vi "Struct Fill Cluster By Items Record.vi"(7 "reinit cluster to default (false)":bool, 8 "error in":errorcluster, 9 "data start offset (0)":i32, 10 "data in":u8[](array[numeric])=[9, 0, 0, 0, 15, 0, 0, 0, 1, 78, 0, 1, 0, 0, 0, 1, 0, 0, 0, 1, 0, 0, 0, 43, 0, 0, 0, 1, 97, 3, 1, 0, 0, 0, 4, 0, 0, 0, 0, 0, 0, 0, 0, 0, 240, 63, 0, 0, 0, 0, 0, 0, 0, 64, 0, 0, 0, 0, 0, 0, 8, 64, 0, 0, 0, 0, 0, 0, 16, 64, 43, 0, 0, 0, 1, 66, 3, 2, 0, 0, 0, 2, 0, 0, 0, 0, 0, 0, 0, 0, 0, 240, 63, 0, 0, 0, 0, 0, 0, 8, 64, 0, 0, 0, 0, 0, 0, 0, 64, 0, 0, 0, 0, 0, 0, 16, 64, 22, 0, 0, 0, 3, 115, 116, 114, 4, 1, 0, 0, 0, 9, 0, 0, 0, 100, 118, 101, 32, 104, 111, 118, 110, 111, 44, 0, 0, 0, 2, 99, 97, 131, 2, 0, 0, 0, 1, 0, 0, 0, 0, 0, 0, 0, 0, 0, 240, 63, 0, 0, 0, 0, 0, 0, 240, 63, 0, 0, 0, 0, 0, 0, 0, 64, 0, 0, 0, 0, 0, 0, 240, 191, 109, 0, 0, 0, 5, 115, 116, 114, 117, 99, 5, 1, 0, 0, 0, 1, 0, 0, 0, 3, 0, 0, 0, 16, 0, 0, 0, 3, 115, 116, 114, 4, 1, 0, 0, 0, 3, 0, 0, 0, 97, 115, 115, 19, 0, 0, 0, 1, 110, 3, 1, 0, 0, 0, 1, 0, 0, 0, 0, 0, 0, 0, 0, 128, 75, 64, 43, 0, 0, 0, 1, 65, 3, 2, 0, 0, 0, 2, 0, 0, 0, 0, 0, 0, 0, 0, 0, 240, 63, 0, 0, 0, 0, 0, 0, 8, 64, 0, 0, 0, 0, 0, 0, 0, 64, 0, 0, 0, 0, 0, 0, 16, 64, 218, 0, 0, 0, 2, 115, 118, 5, 1, 0, 0, 0, 2, 0, 0, 0, 3, 0, 0, 0, 16, 0, 0, 0, 3, 115, 116, 114, 4, 1, 0, 0, 0, 3, 0, 0, 0, 97, 115, 115, 19, 0, 0, 0, 1, 110, 3, 1, 0, 0, 0, 1, 0, 0, 0, 0, 0, 0, 0, 0, 128, 75, 64, 43, 0, 0, 0, 1, 65, 3, 2, 0, 0, 0, 2, 0, 0, 0, 0, 0, 0, 0, 0, 0, 240, 63, 0, 0, 0, 0, 0, 0, 8, 64, 0, 0, 0, 0, 0, 0, 0, 64, 0, 0, 0, 0, 0, 0, 16, 64, 3, 0, 0, 0, 34, 0, 0, 0, 3, 115, 116, 114, 4, 1, 0, 0, 0, 21, 0, 0, 0, 110, 101, 106, 97, 107, 101, 106, 32, 106, 105, 110, 101, 106, 32, 114, 101, 116, 101, 122, 101, 99, 19, 0, 0, 0, 1, 110, 3, 1, 0, 0, 0, 1, 0, 0, 0, 0, 0, 0, 0, 0, 0, 86, 64, 43, 0, 0, 0, 1, 65, 3, 2, 0, 0, 0, 2, 0, 0, 0, 0, 0, 0, 0, 0, 0, 240, 63, 0, 0, 0, 0, 0, 0, 8, 64, 0, 0, 0, 0, 0, 0, 0, 64, 0, 0, 0, 0, 0, 0, 16, 64, 132, 1, 0, 0, 2, 115, 99, 5, 2, 0, 0, 0, 2, 0, 0, 0, 3, 0, 0, 0, 16, 0, 0, 0, 3, 115, 116, 114, 4, 1, 0, 0, 0, 3, 0, 0, 0, 97, 115, 115, 19, 0, 0, 0, 1, 110, 3, 1, 0, 0, 0, 1, 0, 0, 0, 0, 0, 0, 0, 0, 128, 75, 64, 43, 0, 0, 0, 1, 65, 3, 2, 0, 0, 0, 2, 0, 0, 0, 0, 0, 0, 0, 0, 0, 240, 63, 0, 0, 0, 0, 0, 0, 8, 64, 0, 0, 0, 0, 0, 0, 0, 64, 0, 0, 0, 0, 0, 0, 16, 64, 3, 0, 0, 0, 16, 0, 0, 0, 3, 115, 116, 114, 4, 1, 0, 0, 0, 3, 0, 0, 0, 97, 115, 115, 19, 0, 0, 0, 1, 110, 3, 1, 0, 0, 0, 1, 0, 0, 0, 0, 0, 0, 0, 0, 128, 75, 64, 43, 0, 0, 0, 1, 65, 3, 2, 0, 0, 0, 2, 0, 0, 0, 0, 0, 0, 0, 0, 0, 240, 63, 0, 0, 0, 0, 0, 0, 8, 64, 0, 0, 0, 0, 0, 0, 0, 64, 0, 0, 0, 0, 0, 0, 16, 64, 3, 0, 0, 0, 16, 0, 0, 0, 3, 115, 116, 114, 4, 1, 0, 0, 0, 3, 0, 0, 0, 97, 115, 115, 19, 0, 0, 0, 1, 110, 3, 1, 0, 0, 0, 1, 0, 0, 0, 0, 0, 0, 0, 0, 128, 75, 64, 43, 0, 0, 0, 1, 65, 3, 2, 0, 0, 0, 2, 0, 0, 0, 0, 0, 0, 0, 0, 0, 240, 63, 0, 0, 0, 0, 0, 0, 8, 64, 0, 0, 0, 0, 0, 0, 0, 64, 0, 0, 0, 0, 0, 0, 16, 64, 3, 0, 0, 0, 16, 0, 0, 0, 3, 115, 116, 114, 4, 1, 0, 0, 0, 3, 0, 0, 0, 97, 115, 115, 19, 0, 0, 0, 1, 110, 3, 1, 0, 0, 0, 1, 0, 0, 0, 0, 0, 0, 0, 0, 128, 75, 64, 43, 0, 0, 0, 1, 65, 3, 2, 0, 0, 0, 2, 0, 0, 0, 0, 0, 0, 0, 0, 0, 240, 63, 0, 0, 0, 0, 0, 0, 8, 64, 0, 0, 0, 0, 0, 0, 0, 64, 0, 0, 0, 0, 0, 0, 16, 64, 26, 0, 0, 0, 4, 99, 115, 116, 114, 5, 1, 0, 0, 0, 3, 0, 0, 0, 0, 0, 0, 0, 0, 0, 0, 0, 0, 0, 0, 0], 11 "cluster ref (empty)":refnum<vi>) -> (0 "error out":errorcluster, 2 "octave struct out":T1[](array[typedef]), 3 "cluster ref out (copy)":refnum<vi>)   [LabVIEW 2013, in "GOLPI library.lvlib"]
doc: "This VI will use binary struct data generated by GNU Octave GOLPI function 'golpi_conv_struct()'. It will try to assign all elements from the Octave to the elements of matching names in the referenced cluser. Optionally it can reset the cluster default before. If it is called with invalid reference to the cluster it will just parse the binary data and return the items list. The function is recoursive so it should be able to assign clusters within clusters and so on."
uses:
  GOLPI library.lvlib
  Type Definitions/Struct Item Record.ctl
  Type Definitions/Struct Item Types.ctl
  Type Definitions/Custom Error Codes Enum Type Def.vi
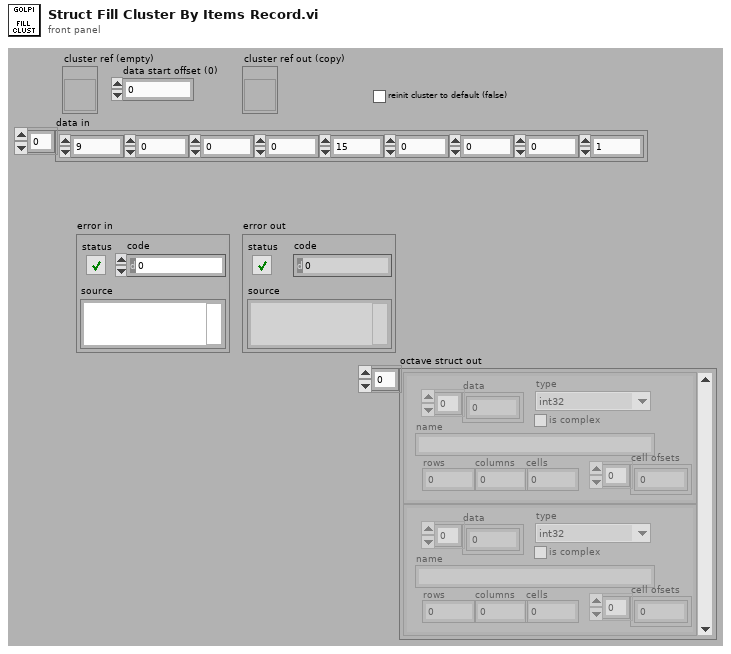
[diagram p1: front panel]
types:
  T1 = typedef "GOLPI library.lvlib/Struct Item Record.ctl" = cluster{"data":u8[], "type":T2, "name":string, "rows":i32, "columns":i32, "cells":i32, "is complex":bool, "cell ofsets":u32[]}
  T2 = typedef "GOLPI library.lvlib/Struct Item Types.ctl" = enum16{"int32", "uint32", "single", "double", "string", "cell array"}
  T3 = typedef "GOLPI library.lvlib/Custom Error Codes Enum Type Def.vi" = enum16{"no error", "00 working directory PAR1 missing", "01 octave binary PAR1 missing", "02 octave report error PAR1", "03 empty output last cmd PAR1", "04 missing temporary file PAR1", "05 pwd PAR 1 not exist", "06 oct package not installed", "10 var PAR1 not string, vect", "11 var PAR1 not num, scal, ~compl", "12 var PAR1 not num, scal, compl", "13 var PAR1 not num, vect, ~compl", "14 var PAR1 not num, vect, compl", "15 var PAR1 not num, mat, ~compl", "16 var PAR1 not num, mat, ~compl", "30 read timeout", "60 bitstream transport failed", "61 bitstream decode error PAR1", "62 bitstream cannot be set", "70 struct transfer not possible", "80 struct: cluster elem. PAR1 not implem.", "81 struct: structure field PAR1 not implem.", "82 struct: size mismatch of PAR1", "83 struct: type mismatch of PAR1", "98 internal error", "99 not finished"}
  T4 = enum16{"big-endian, network order", "native, host order", "little-endian"}
  T5 = typedef "GOLPI library.lvlib/Struct Data Types.ctl" = enum16{"n/a", "Real", "Complex", "String/path", "Cluster", "Bool"}
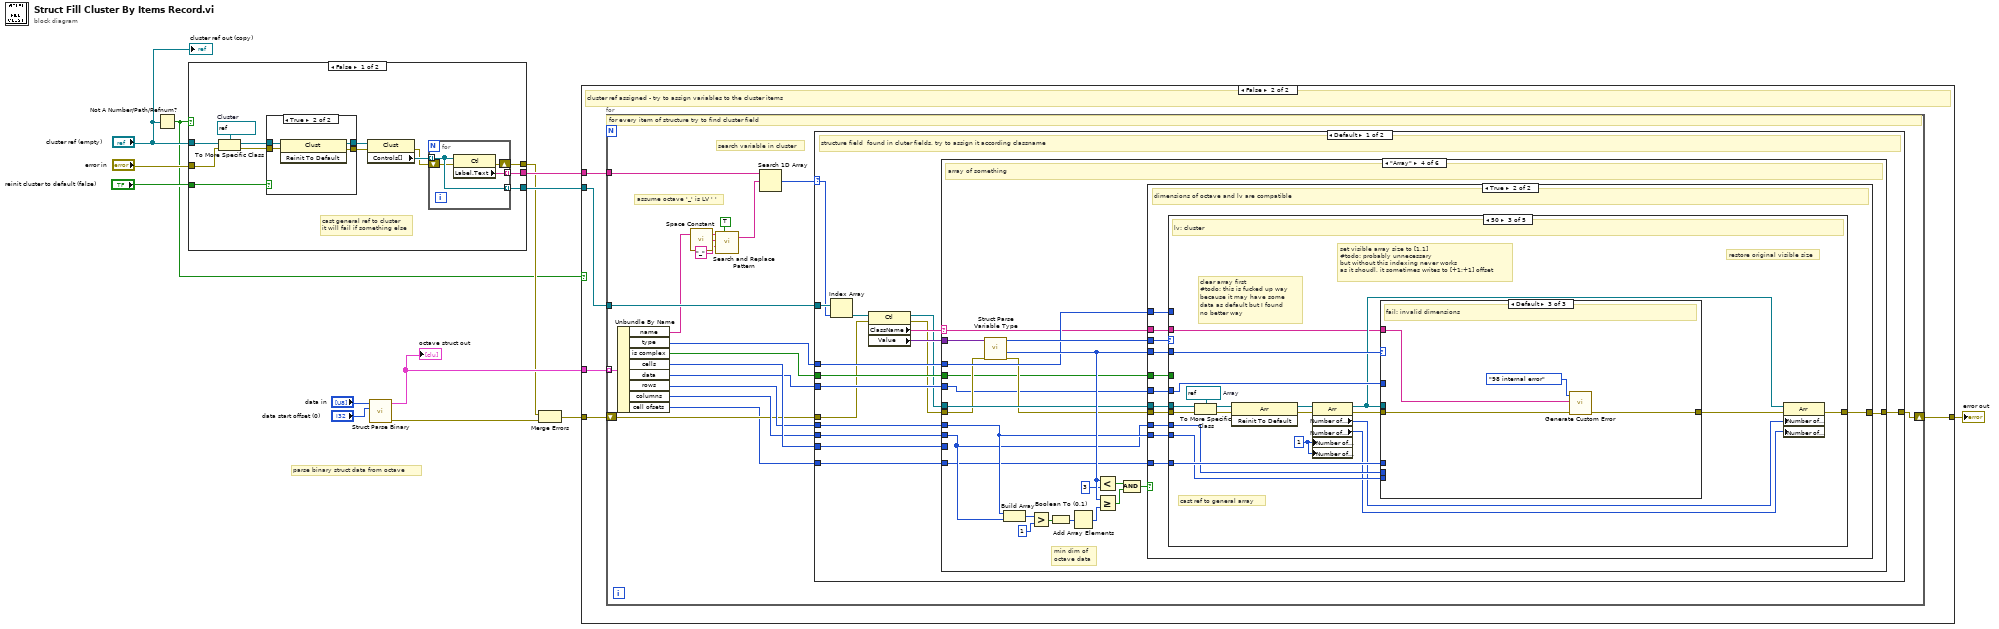
[diagram p0: block diagram]
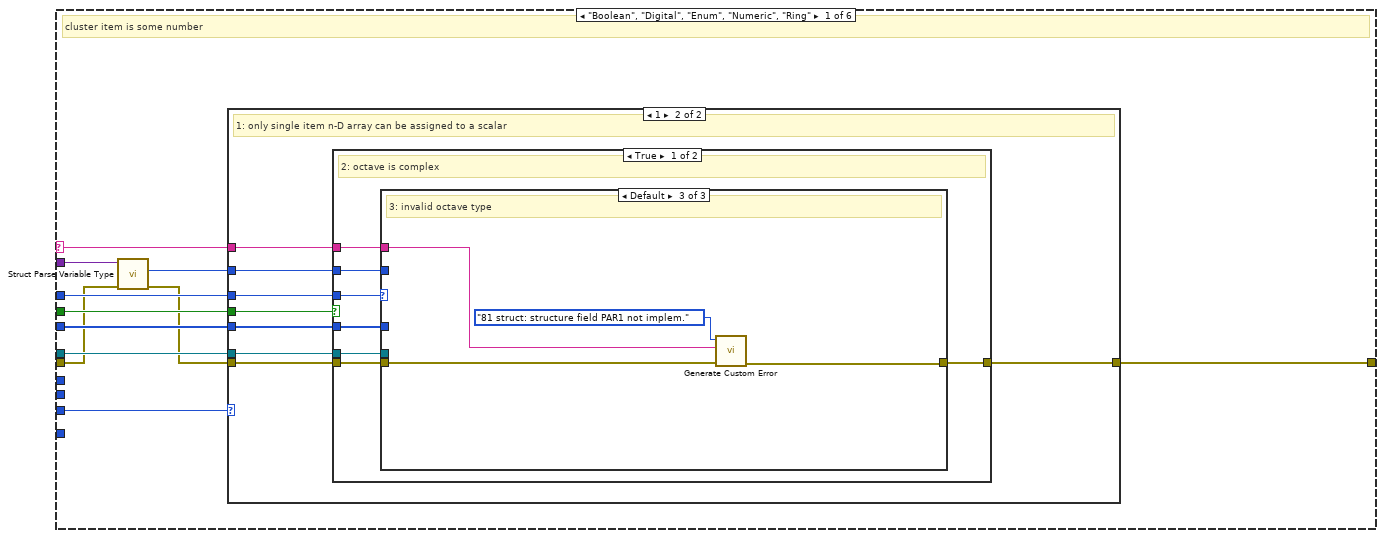
[diagram p3: hidden frame]
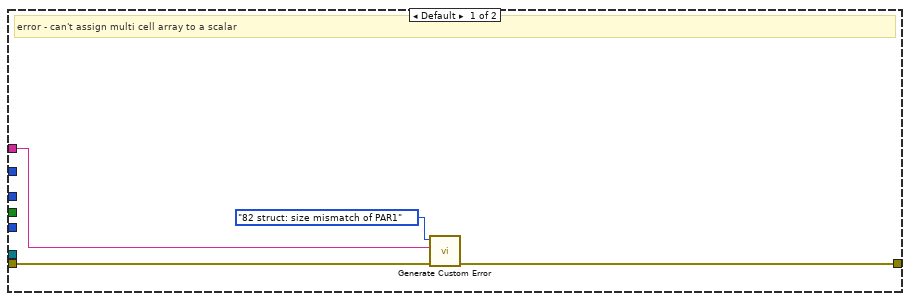
[diagram p4: hidden frame]
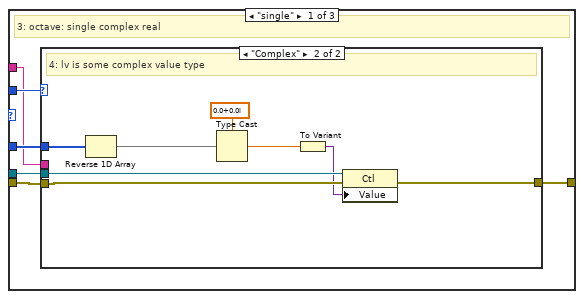
[diagram p5: hidden frame]
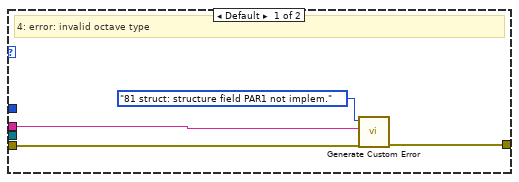
[diagram p6: hidden frame]
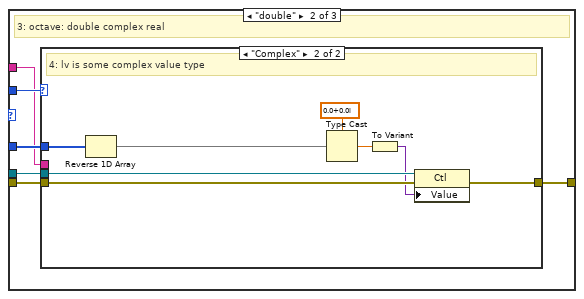
[diagram p7: hidden frame]
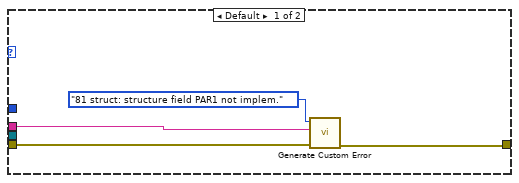
[diagram p8: hidden frame]
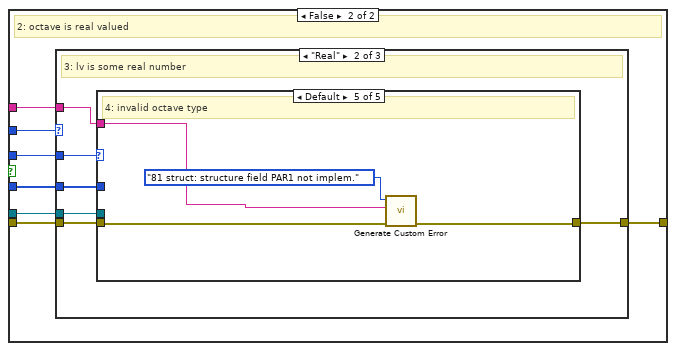
[diagram p9: hidden frame]
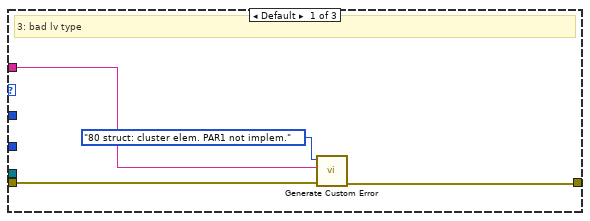
[diagram p10: hidden frame]
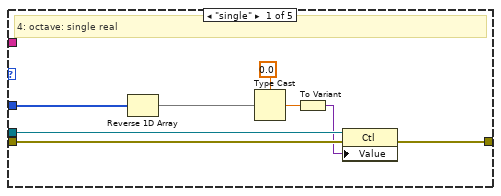
[diagram p11: hidden frame]
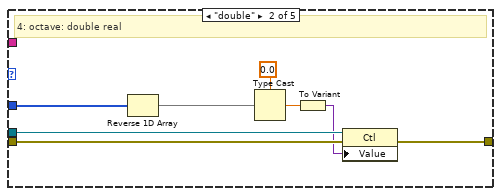
[diagram p12: hidden frame]
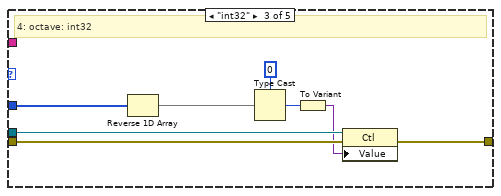
[diagram p13: hidden frame]
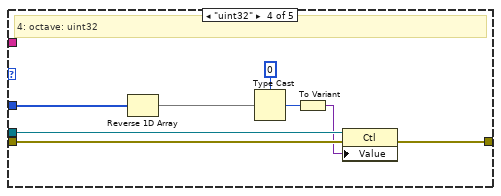
[diagram p14: hidden frame]
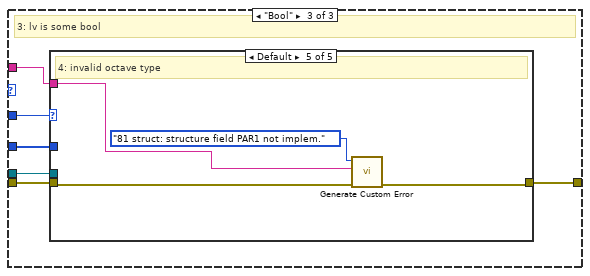
[diagram p15: hidden frame]
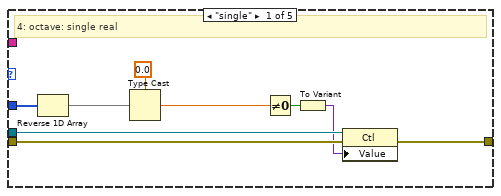
[diagram p16: hidden frame]
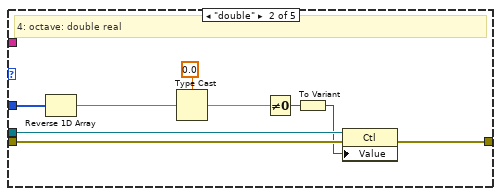
[diagram p17: hidden frame]
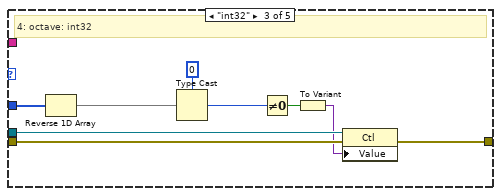
[diagram p18: hidden frame]
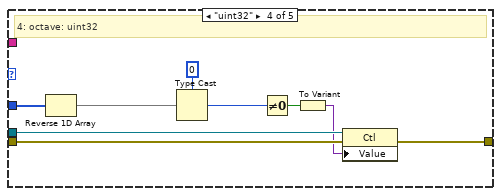
[diagram p19: hidden frame]
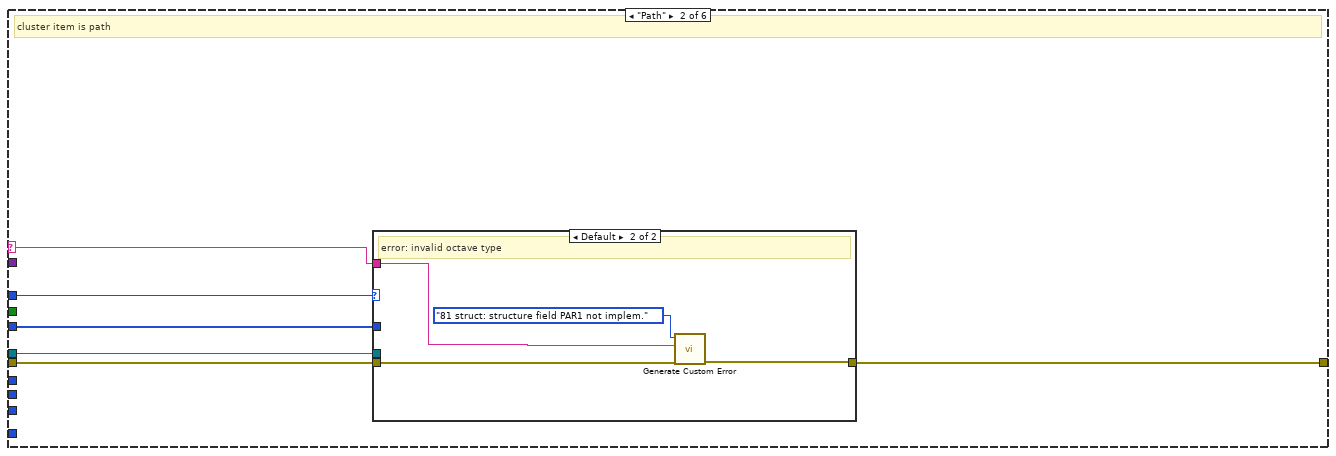
[diagram p20: hidden frame]
diagram:
  # "parse binary struct data from octave"
  n1 = Not A Number/Path/Refnum?(number/path/refnum="cluster ref (empty)") -> (NaN/Path/Refnum?=w1:bool)
  n2 = case shown="False" w1 {
    tunnel: [w25 _] -> w11
    tunnel: [w24 _] -> w10
    tunnel: "error in" -> [w22 w37]
    tunnel: "cluster ref (empty)" -> [w15 _]
    tunnel: "reinit cluster to default (false)" -> [w17 _]
    tunnel: [w14 w37] -> w4
    frame False {
      w23 = refnum<vi> refnum  # Cluster
      # "cast general ref to cluster\nit will fail if something else"
      n3 = To More Specific Class(target class=w23, reference=w15, error in=w22) -> (specific class reference=w19:refnum<vi>, error out=w18:errorcluster)
      n4 = case shown="True" w17 {
        tunnel: [w28 w32] -> w21
        tunnel: [w27 w31] -> w20
        tunnel: w19 -> [w27 w30]
        tunnel: w18 -> [w28 w29]
        frame False {
        }
        frame True {
          n5 = invoke class="Clust" method="Reinit To Default"(reference=w30, error in=w29) -> (reference out=w31:refnum<vi>, error out=w32:errorcluster)  [unwired: 1 in, 1 out]
        }
      }
      n6 = property class="Clust"(reference=w20, error in=w21) -> (error out=w16:errorcluster, "Controls[]"=w26:refnum<vi>[])  [unwired: 1 out]
      n7 = for {
        tunnel: w26 -> [w35] mode=indexing
        tunnel: [w36] -> w25 mode=indexing
        tunnel: [w35] -> w24 mode=indexing
        shift-right: [w33] -> w14
        shift-left: w16 -> [w34]
        n8 = property class="Ctl"(reference=w35, error in=w34) -> (error out=w33:errorcluster, "Label.Text"=w36:string)  [unwired: 1 out]
      }
    }
    frame True {
    }
  }
  n9 = call "Struct Parse Binary.vi"("data start offset (0)"="data start offset (0)", "data in"="data in") -> ("error out"=w3:errorcluster, "struct items"=w12:T1[])  [unwired: 8 in]
  "octave struct out" <- w12
  n10 = Merge Errors(w4, w3) -> (w2:errorcluster)
  n11 = case shown="False" w1 {
    tunnel: w12 -> [_ w43]
    tunnel: w11 -> [_ w42]
    tunnel: w10 -> [_ w41]
    tunnel: [w38 w40] -> w9
    tunnel: w2 -> [w38 w39]
    frame True {
      # "no cluster ref assigned - skip assigning, just parse struct"
    }
    frame False {
      # "cluster ref assigned - try to assign variables to the cluster items"
      n12 = for {
        tunnel: w43 -> [w61] mode=indexing
        tunnel: w42 -> [w60]
        tunnel: w41 -> [w59]
        shift-right: [w52] -> w40
        shift-left: w39 -> [w51]
        # "assume octave '_' is LV ' '"
        # "search variable in cluster"
        # "for every item of structure try to find cluster field"
        n13 = Unbundle By Name(w61) -> ("name"=w48:string, "type"=w58:T2, "is complex"=w57:bool, "cells"=w56:i32, "data"=w55:u8[], "rows"=w54:i32, "columns"=w53:i32, "cell ofsets"=w50:u32[])
        n14 = call <vilib>:"Space Constant.vi"() -> ("String"=w44:string)
        n15 = call <vilib>:"Search and Replace Pattern.vi"("string"=w48, "regular expression (\"\")"="_", "replace string (\"\")"=w44, "replace all? (F)"=TRUE) -> ("result string"=w47:string)  [unwired: 1 in, 1 out]
        n16 = Search 1D Array(1D array=w60, element=w47) -> (index of element=w49:i32)  [unwired: 1 in]
        n17 = case shown="Default" w49 {
          selector: w49 -> [w76 _]
          tunnel: w59 -> [w77 _]
          tunnel: w58 -> [w72 _]
          tunnel: w57 -> [w71 _]
          tunnel: w56 -> [w70 _]
          tunnel: w55 -> [w69 _]
          tunnel: w54 -> [w66 _]
          tunnel: w53 -> [w65 _]
          tunnel: [w64 w696] -> w52
          tunnel: w51 -> [w63 w696]
          tunnel: w50 -> [w62 _]
          frame Default {
            # "structure field  found in cluter fields, try to assign it according classname"
            n18 = Index Array(array=w77, index=w76) -> (element=w75:refnum<vi>)
            n19 = property class="Ctl"(reference=w75, error in=w63) -> (reference out=w68:refnum<vi>, error out=w67:errorcluster, "ClassName"=w74:string, "Value"=w73:variant)
            n20 = case shown="\"Array\"" w74 {
              selector: w74 -> [w78 w247 w264 w280 _ w694]
              tunnel: w73 -> [w88 _ _ w282 _ _]
              tunnel: w72 -> [w87 w252 w269 w289 w678 _]
              tunnel: w71 -> [w83 _ _ w286 _ _]
              tunnel: w70 -> [w84 _ _ _ w680 _]
              tunnel: w69 -> [w86 w251 w268 w285 w672 _]
              tunnel: w68 -> [w82 w250 w267 w291 w673 _]
              tunnel: w67 -> [w80 w249 w266 w288 w681 w693]
              tunnel: [w81 w248 w265 w292 w671 w692] -> w64
              tunnel: w66 -> [_ _ _ w284 _ _]
              tunnel: w65 -> [_ _ _ w283 _ _]
              tunnel: w62 -> [_ _ _ w281 _ _]
              frame "Boolean", "Digital", "Enum", "Numeric", "Ring" {
                # "cluster item is some number"
                n21 = call "Struct Parse Variable Type.vi"("error in"=w80, "variant in"=w88) -> ("error out"=w79:errorcluster, "data type"=w85:T5)  [unwired: 6 in, 2 out]
                n22 = case shown="1" w84 {
                  tunnel: w87 -> [_ w100]
                  tunnel: w86 -> [_ w99]
                  tunnel: w85 -> [_ w98]
                  tunnel: w83 -> [_ w97]
                  tunnel: w82 -> [_ w96]
                  tunnel: w79 -> [w91 w95]
                  tunnel: [w90 w94] -> w81
                  tunnel: w78 -> [w89 w93]
                  frame Default {
                    # "error - can't assign multi cell array to a scalar"
                    n23 = call "Generate Custom Error.vi"("error in"=w91, "PAR1"=w89, "GOLPI error"=Custom_Error_Codes_Enum_Type_Def.vi."82 struct: size mismatch of PAR1") -> ("error out"=w90:errorcluster)  [unwired: 8 in]
                  }
                  frame 1 {
                    # "1: only single item n-D array can be assigned to a scalar"
                    n24 = case shown="True" w97 {
                      tunnel: w100 -> [w107 w154]
                      tunnel: w99 -> [w106 w153]
                      tunnel: w98 -> [w105 w149]
                      tunnel: w96 -> [w104 w152]
                      tunnel: w95 -> [w103 w151]
                      tunnel: [w102 w150] -> w94
                      tunnel: w93 -> [w101 w148]
                      frame True {
                        # "2: octave is complex"
                        n25 = case shown="Default" w107 {
                          tunnel: w106 -> [w112 w130 _]
                          tunnel: w105 -> [w113 w131 _]
                          tunnel: w104 -> [w111 w129 _]
                          tunnel: w103 -> [w110 w128 w146]
                          tunnel: [w109 w127 w145] -> w102
                          tunnel: w101 -> [w108 w126 w144]
                          frame "single" {
                            # "3: octave: single complex real"
                            n26 = case shown="\"Complex\"" w113 {
                              tunnel: w112 -> [_ w125]
                              tunnel: w111 -> [_ w122]
                              tunnel: w110 -> [w116 w121]
                              tunnel: [w115 w118] -> w109
                              tunnel: w108 -> [w114 _]
                              frame Default {
                                # "4: error: invalid octave type"
                                n27 = call "Generate Custom Error.vi"("error in"=w116, "PAR1"=w114, "GOLPI error"=Custom_Error_Codes_Enum_Type_Def.vi."81 struct: structure field PAR1 not implem.") -> ("error out"=w115:errorcluster)  [unwired: 8 in]
                              }
                              frame "Complex" {
                                # "4: lv is some complex value type"
                                n28 = Reverse 1D Array(array=w125) -> (reversed array=w124:u8[])
                                n29 = Type Cast(type=csg 0.0+0.0i, x=w124) -> (*(type *) &x=w120:csg)
                                n30 = To Variant(anything=w120) -> (Variant=w119:variant)
                                n31 = property class="Ctl"(reference=w122, error in=w121, "Value"=w119) -> (error out=w118:errorcluster)  [unwired: 1 out]
                              }
                            }
                          }
                          frame "double" {
                            # "3: octave: double complex real"
                            n32 = case shown="\"Complex\"" w131 {
                              tunnel: w130 -> [_ w143]
                              tunnel: w129 -> [_ w140]
                              tunnel: w128 -> [w134 w139]
                              tunnel: [w133 w136] -> w127
                              tunnel: w126 -> [w132 _]
                              frame Default {
                                n33 = call "Generate Custom Error.vi"("error in"=w134, "PAR1"=w132, "GOLPI error"=Custom_Error_Codes_Enum_Type_Def.vi."81 struct: structure field PAR1 not implem.") -> ("error out"=w133:errorcluster)  [unwired: 8 in]
                              }
                              frame "Complex" {
                                # "4: lv is some complex value type"
                                n34 = Reverse 1D Array(array=w143) -> (reversed array=w142:u8[])
                                n35 = Type Cast(type=cdb 0.0+0.0i, x=w142) -> (*(type *) &x=w138:cdb)
                                n36 = To Variant(anything=w138) -> (Variant=w137:variant)
                                n37 = property class="Ctl"(reference=w140, error in=w139, "Value"=w137) -> (error out=w136:errorcluster)  [unwired: 1 out]
                              }
                            }
                          }
                          frame Default {
                            # "3: invalid octave type"
                            n38 = call "Generate Custom Error.vi"("error in"=w146, "PAR1"=w144, "GOLPI error"=Custom_Error_Codes_Enum_Type_Def.vi."81 struct: structure field PAR1 not implem.") -> ("error out"=w145:errorcluster)  [unwired: 8 in]
                          }
                        }
                      }
                      frame False {
                        # "2: octave is real valued"
                        n39 = case shown="\"Real\"" w149 {
                          tunnel: w154 -> [_ w164 w206]
                          tunnel: w153 -> [_ w163 w205]
                          tunnel: w152 -> [_ w162 w204]
                          tunnel: w151 -> [w157 w161 w203]
                          tunnel: [w156 w160 w202] -> w150
                          tunnel: w148 -> [w155 w159 w201]
                          frame Default {
                            # "3: bad lv type"
                            n40 = call "Generate Custom Error.vi"("error in"=w157, "PAR1"=w155, "GOLPI error"=Custom_Error_Codes_Enum_Type_Def.vi."80 struct: cluster elem. PAR1 not implem.") -> ("error out"=w156:errorcluster)  [unwired: 8 in]
                          }
                          frame "Real" {
                            # "3: lv is some real number"
                            n41 = case shown="Default" w164 {
                              tunnel: w163 -> [w172 w180 w188 w196 _]
                              tunnel: w162 -> [w171 w179 w187 w195 _]
                              tunnel: w161 -> [w170 w178 w186 w194 w199]
                              tunnel: [w169 w177 w185 w193 w198] -> w160
                              tunnel: w159 -> [_ _ _ _ w197]
                              frame "single" {
                                # "4: octave: single real"
                                n42 = Reverse 1D Array(array=w172) -> (reversed array=w168:u8[])
                                n43 = Type Cast(type=sgl 0.0, x=w168) -> (*(type *) &x=w166:sgl)
                                n44 = To Variant(anything=w166) -> (Variant=w165:variant)
                                n45 = property class="Ctl"(reference=w171, error in=w170, "Value"=w165) -> (error out=w169:errorcluster)  [unwired: 1 out]
                              }
                              frame "double" {
                                # "4: octave: double real"
                                n46 = Reverse 1D Array(array=w180) -> (reversed array=w176:u8[])
                                n47 = Type Cast(type=0.0, x=w176) -> (*(type *) &x=w174:dbl)
                                n48 = To Variant(anything=w174) -> (Variant=w173:variant)
                                n49 = property class="Ctl"(reference=w179, error in=w178, "Value"=w173) -> (error out=w177:errorcluster)  [unwired: 1 out]
                              }
                              frame "int32" {
                                # "4: octave: int32"
                                n50 = Reverse 1D Array(array=w188) -> (reversed array=w184:u8[])
                                n51 = Type Cast(type=0, x=w184) -> (*(type *) &x=w182:i32)
                                n52 = To Variant(anything=w182) -> (Variant=w181:variant)
                                n53 = property class="Ctl"(reference=w187, error in=w186, "Value"=w181) -> (error out=w185:errorcluster)  [unwired: 1 out]
                              }
                              frame "uint32" {
                                # "4: octave: uint32"
                                n54 = Reverse 1D Array(array=w196) -> (reversed array=w192:u8[])
                                n55 = Type Cast(type=u32 0, x=w192) -> (*(type *) &x=w190:u32)
                                n56 = To Variant(anything=w190) -> (Variant=w189:variant)
                                n57 = property class="Ctl"(reference=w195, error in=w194, "Value"=w189) -> (error out=w193:errorcluster)  [unwired: 1 out]
                              }
                              frame Default {
                                # "4: invalid octave type"
                                n58 = call "Generate Custom Error.vi"("error in"=w199, "PAR1"=w197, "GOLPI error"=Custom_Error_Codes_Enum_Type_Def.vi."81 struct: structure field PAR1 not implem.") -> ("error out"=w198:errorcluster)  [unwired: 8 in]
                              }
                            }
                          }
                          frame "Bool" {
                            # "3: lv is some bool"
                            n59 = case shown="Default" w206 {
                              tunnel: w205 -> [w215 w224 w233 w242 _]
                              tunnel: w204 -> [w214 w223 w232 w241 _]
                              tunnel: w203 -> [w213 w222 w231 w240 w245]
                              tunnel: [w212 w221 w230 w239 w244] -> w202
                              tunnel: w201 -> [_ _ _ _ w243]
                              frame "single" {
                                # "4: octave: single real"
                                n60 = Reverse 1D Array(array=w215) -> (reversed array=w211:u8[])
                                n61 = Type Cast(type=sgl 0.0, x=w211) -> (*(type *) &x=w209:sgl)
                                n62 = Not Equal To 0?(x=w209) -> (x != 0?=w207:bool)
                                n63 = To Variant(anything=w207) -> (Variant=w208:variant)
                                n64 = property class="Ctl"(reference=w214, error in=w213, "Value"=w208) -> (error out=w212:errorcluster)  [unwired: 1 out]
                              }
                              frame "double" {
                                # "4: octave: double real"
                                n65 = Reverse 1D Array(array=w224) -> (reversed array=w220:u8[])
                                n66 = Type Cast(type=0.0, x=w220) -> (*(type *) &x=w218:dbl)
                                n67 = Not Equal To 0?(x=w218) -> (x != 0?=w216:bool)
                                n68 = To Variant(anything=w216) -> (Variant=w217:variant)
                                n69 = property class="Ctl"(reference=w223, error in=w222, "Value"=w217) -> (error out=w221:errorcluster)  [unwired: 1 out]
                              }
                              frame "int32" {
                                # "4: octave: int32"
                                n70 = Reverse 1D Array(array=w233) -> (reversed array=w229:u8[])
                                n71 = Type Cast(type=0, x=w229) -> (*(type *) &x=w227:i32)
                                n72 = Not Equal To 0?(x=w227) -> (x != 0?=w225:bool)
                                n73 = To Variant(anything=w225) -> (Variant=w226:variant)
                                n74 = property class="Ctl"(reference=w232, error in=w231, "Value"=w226) -> (error out=w230:errorcluster)  [unwired: 1 out]
                              }
                              frame "uint32" {
                                # "4: octave: uint32"
                                n75 = Reverse 1D Array(array=w242) -> (reversed array=w238:u8[])
                                n76 = Type Cast(type=u32 0, x=w238) -> (*(type *) &x=w236:u32)
                                n77 = Not Equal To 0?(x=w236) -> (x != 0?=w234:bool)
                                n78 = To Variant(anything=w234) -> (Variant=w235:variant)
                                n79 = property class="Ctl"(reference=w241, error in=w240, "Value"=w235) -> (error out=w239:errorcluster)  [unwired: 1 out]
                              }
                              frame Default {
                                # "4: invalid octave type"
                                n80 = call "Generate Custom Error.vi"("error in"=w245, "PAR1"=w243, "GOLPI error"=Custom_Error_Codes_Enum_Type_Def.vi."81 struct: structure field PAR1 not implem.") -> ("error out"=w244:errorcluster)  [unwired: 8 in]
                              }
                            }
                          }
                        }
                      }
                    }
                  }
                }
              }
              frame "Path" {
                # "cluster item is path"
                n81 = case shown="Default" w252 {
                  tunnel: w251 -> [w255 _]
                  tunnel: w250 -> [w259 _]
                  tunnel: w249 -> [w258 w262]
                  tunnel: [w257 w261] -> w248
                  tunnel: w247 -> [_ w260]
                  frame "string" {
                    # "octave: string"
                    n82 = Byte Array To String(unsigned byte array=w255) -> (string=w254:string)
                    n83 = String To Path(string=w254) -> (path=w253:path)
                    n84 = To Variant(anything=w253) -> (Variant=w256:variant)
                    n85 = property class="Ctl"(reference=w259, error in=w258, "Value"=w256) -> (error out=w257:errorcluster)  [unwired: 1 out]
                  }
                  frame Default {
                    # "error: invalid octave type"
                    n86 = call "Generate Custom Error.vi"("error in"=w262, "PAR1"=w260, "GOLPI error"=Custom_Error_Codes_Enum_Type_Def.vi."81 struct: structure field PAR1 not implem.") -> ("error out"=w261:errorcluster)  [unwired: 8 in]
                  }
                }
              }
              frame "ComboBox", "DAQmxName", "IVILogicalName", "IVIResourceName", "String", "VISAResourceName" {
                # "cluster item is some string type"
                n87 = case shown="Default" w269 {
                  tunnel: w268 -> [w271 _]
                  tunnel: w267 -> [w275 _]
                  tunnel: w266 -> [w274 w278]
                  tunnel: [w273 w277] -> w265
                  tunnel: w264 -> [_ w276]
                  frame "string" {
                    # "octave: string"
                    n88 = Byte Array To String(unsigned byte array=w271) -> (string=w270:string)
                    n89 = To Variant(anything=w270) -> (Variant=w272:variant)
                    n90 = property class="Ctl"(reference=w275, error in=w274, "Value"=w272) -> (error out=w273:errorcluster)  [unwired: 1 out]
                  }
                  frame Default {
                    # "error: invalid octave type"
                    n91 = call "Generate Custom Error.vi"("error in"=w278, "PAR1"=w276, "GOLPI error"=Custom_Error_Codes_Enum_Type_Def.vi."81 struct: structure field PAR1 not implem.") -> ("error out"=w277:errorcluster)  [unwired: 8 in]
                  }
                }
              }
              frame "Array" {
                # "min dim of\noctave data"
                # "array of something"
                n92 = call "Struct Parse Variable Type.vi"("error in"=w288, "variant in"=w282) -> ("error out"=w287:errorcluster, "array dims"=w297:i16, "type id"=w290:i16)  [unwired: 6 in, 1 out]
                n93 = Build Array(w284, w283) -> (w302:i32[])
                n94 = Greater?(x=w302, y=1) -> (0:w300:bool[])
                n95 = Boolean To (0,1)(Boolean=w300) -> (0, 1=w299:i16[])
                n96 = Add Array Elements(numeric array=w299) -> (sum=w298:i16)
                n97 = Less?(x=w297, y=i16 3) -> (x < y?=w295:bool)
                n98 = Greater Or Equal?(x=w297, y=w298) -> (x >= y?=w294:bool)
                n99 = Compound Arithmetic op=AND(w295, w294) -> (w293:bool)
                n100 = case shown="True" w293 {
                  tunnel: w290 -> [_ w318]
                  tunnel: w297 -> [_ w317]
                  tunnel: [w304 w311] -> w292
                  tunnel: w287 -> [w305 w315]
                  tunnel: w291 -> [_ w314]
                  tunnel: w289 -> [_ w316]
                  tunnel: w286 -> [_ w313]
                  tunnel: w285 -> [_ w312]
                  tunnel: w283 -> [_ w310]
                  tunnel: w284 -> [_ w309]
                  tunnel: w281 -> [_ w308]
                  tunnel: w280 -> [w303 w307]
                  frame False {
                    # "incompatible lv and octave dims"
                    n101 = call "Generate Custom Error.vi"("error in"=w305, "PAR1"=w303, "GOLPI error"=Custom_Error_Codes_Enum_Type_Def.vi."82 struct: size mismatch of PAR1") -> ("error out"=w304:errorcluster)  [unwired: 8 in]
                  }
                  frame True {
                    # "dimensions of octave and lv are compatible"
                    n102 = case shown="50" w318 {
                      selector: w318 -> [_ _ _ w575 _]
                      tunnel: w317 -> [w322 w437 w510 w581 _]
                      tunnel: w316 -> [w328 w443 _ _ _]
                      tunnel: w315 -> [w327 w442 w523 w585 w668]
                      tunnel: w314 -> [w326 w441 w524 w586 _]
                      tunnel: w313 -> [w325 w440 _ _ _]
                      tunnel: w312 -> [w324 w439 w521 w583 _]
                      tunnel: [w323 w438 w511 w574 w669] -> w311
                      tunnel: w310 -> [w321 w436 w518 w578 _]
                      tunnel: w309 -> [w320 w435 w519 w577 _]
                      tunnel: w308 -> [_ _ w520 w582 _]
                      tunnel: w307 -> [w319 w434 w505 _ w667]
                      frame 1..11, 21..23 {
                        # "lv: real numerics"
                        n103 = case shown="False" w325 {
                          tunnel: w328 -> [w337 _]
                          tunnel: w327 -> [w336 w432]
                          tunnel: w326 -> [w333 _]
                          tunnel: w324 -> [w335 _]
                          tunnel: [w334 w431] -> w323
                          tunnel: w322 -> [w332 _]
                          tunnel: w321 -> [w331 _]
                          tunnel: w320 -> [w330 _]
                          tunnel: w319 -> [w329 w430]
                          frame False {
                            # "octave: real"
                            n104 = case shown="Default" w337 {
                              tunnel: w336 -> [w340 w362 w384 w406 w428]
                              tunnel: w335 -> [w339 w361 w383 w405 _]
                              tunnel: [w347 w369 w391 w413 w427] -> w334
                              tunnel: w333 -> [w348 w370 w392 w414 _]
                              tunnel: w332 -> [w345 w367 w389 w411 _]
                              tunnel: w331 -> [w343 w365 w387 w409 _]
                              tunnel: w330 -> [w342 w364 w386 w408 _]
                              tunnel: w329 -> [_ _ _ _ w426]
                              frame "int32" {
                                # "octave: int32 array"
                                n105 = Byte Array To String(unsigned byte array=w339) -> (string=w338:string)
                                n106 = Unflatten From String(type=i32[] [], binary string=w338, data includes array or string size? (T)=FALSE ("prepend array or string size? (T)"), byte order (0:big-endian, network order)=T4."little-endian", error in (no error)=w340) -> (value=w346:i32[], error out=w349:errorcluster)  [unwired: 1 out]
                                n107 = case shown="2" w345 {
                                tunnel: w346 -> [w352 w359]
                                tunnel: [w353 w357] -> w344
                                tunnel: w343 -> [_ w356]
                                tunnel: w342 -> [_ w355]
                                frame Default {
                                # "1D"
                                n108 = To Variant(anything=w352) -> (Variant=w353:variant)
                                }
                                frame 2 {
                                # "2D"
                                n109 = Reshape Array(w359, w356, w355) -> (w358:i32[][])
                                n110 = Transpose 2D Array(2D array=w358) -> (transposed array=w354:i32[][])
                                n111 = To Variant(anything=w354) -> (Variant=w357:variant)
                                }
                                }
                                n112 = property class="Ctl"(reference=w348, error in=w349, "Value"=w344) -> (error out=w347:errorcluster)  [unwired: 1 out]
                              }
                              frame "uint32" {
                                # "octave: uint32 array"
                                n113 = Byte Array To String(unsigned byte array=w361) -> (string=w360:string)
                                n114 = Unflatten From String(type=u32[] [], binary string=w360, data includes array or string size? (T)=FALSE ("prepend array or string size? (T)"), byte order (0:big-endian, network order)=T4."little-endian", error in (no error)=w362) -> (value=w368:u32[], error out=w371:errorcluster)  [unwired: 1 out]
                                n115 = case shown="2" w367 {
                                tunnel: w368 -> [w374 w381]
                                tunnel: [w375 w379] -> w366
                                tunnel: w365 -> [_ w378]
                                tunnel: w364 -> [_ w377]
                                frame Default {
                                # "1D"
                                n116 = To Variant(anything=w374) -> (Variant=w375:variant)
                                }
                                frame 2 {
                                # "2D"
                                n117 = Reshape Array(w381, w378, w377) -> (w380:u32[][])
                                n118 = Transpose 2D Array(2D array=w380) -> (transposed array=w376:u32[][])
                                n119 = To Variant(anything=w376) -> (Variant=w379:variant)
                                }
                                }
                                n120 = property class="Ctl"(reference=w370, error in=w371, "Value"=w366) -> (error out=w369:errorcluster)  [unwired: 1 out]
                              }
                              frame "single" {
                                # "octave: single real array"
                                n121 = Byte Array To String(unsigned byte array=w383) -> (string=w382:string)
                                n122 = Unflatten From String(type=sgl[] [], binary string=w382, data includes array or string size? (T)=FALSE ("prepend array or string size? (T)"), byte order (0:big-endian, network order)=T4."little-endian", error in (no error)=w384) -> (value=w390:sgl[], error out=w393:errorcluster)  [unwired: 1 out]
                                n123 = case shown="2" w389 {
                                tunnel: w390 -> [w396 w403]
                                tunnel: [w397 w401] -> w388
                                tunnel: w387 -> [_ w400]
                                tunnel: w386 -> [_ w399]
                                frame Default {
                                # "1D"
                                n124 = To Variant(anything=w396) -> (Variant=w397:variant)
                                }
                                frame 2 {
                                # "2D"
                                n125 = Reshape Array(w403, w400, w399) -> (w402:sgl[][])
                                n126 = Transpose 2D Array(2D array=w402) -> (transposed array=w398:sgl[][])
                                n127 = To Variant(anything=w398) -> (Variant=w401:variant)
                                }
                                }
                                n128 = property class="Ctl"(reference=w392, error in=w393, "Value"=w388) -> (error out=w391:errorcluster)  [unwired: 1 out]
                              }
                              frame "double" {
                                # "octave: double real array"
                                n129 = Byte Array To String(unsigned byte array=w405) -> (string=w404:string)
                                n130 = Unflatten From String(type=dbl[] [], binary string=w404, data includes array or string size? (T)=FALSE ("prepend array or string size? (T)"), byte order (0:big-endian, network order)=T4."little-endian", error in (no error)=w406) -> (value=w412:dbl[], error out=w415:errorcluster)  [unwired: 1 out]
                                n131 = case shown="2" w411 {
                                tunnel: w412 -> [w418 w425]
                                tunnel: [w419 w423] -> w410
                                tunnel: w409 -> [_ w422]
                                tunnel: w408 -> [_ w421]
                                frame Default {
                                # "1D"
                                n132 = To Variant(anything=w418) -> (Variant=w419:variant)
                                }
                                frame 2 {
                                # "2D"
                                n133 = Reshape Array(w425, w422, w421) -> (w424:dbl[][])
                                n134 = Transpose 2D Array(2D array=w424) -> (transposed array=w420:dbl[][])
                                n135 = To Variant(anything=w420) -> (Variant=w423:variant)
                                }
                                }
                                n136 = property class="Ctl"(reference=w414, error in=w415, "Value"=w410) -> (error out=w413:errorcluster)  [unwired: 1 out]
                              }
                              frame Default {
                                # "error: unknown"
                                n137 = call "Generate Custom Error.vi"("error in"=w428, "PAR1"=w426, "GOLPI error"=Custom_Error_Codes_Enum_Type_Def.vi."98 internal error") -> ("error out"=w427:errorcluster)  [unwired: 8 in]
                              }
                            }
                          }
                          frame True {
                            # "not allowed complexes"
                            n138 = call "Generate Custom Error.vi"("error in"=w432, "PAR1"=w430, "GOLPI error"=Custom_Error_Codes_Enum_Type_Def.vi."83 struct: type mismatch of PAR1") -> ("error out"=w431:errorcluster)  [unwired: 8 in]
                          }
                        }
                      }
                      frame 12..14 {
                        # "lv: complex numerics"
                        n139 = case shown="True" w440 {
                          tunnel: w443 -> [w452 _]
                          tunnel: w442 -> [w451 w503]
                          tunnel: w441 -> [w448 _]
                          tunnel: w439 -> [w450 _]
                          tunnel: [w449 w502] -> w438
                          tunnel: w437 -> [w447 _]
                          tunnel: w436 -> [w446 _]
                          tunnel: w435 -> [w445 _]
                          tunnel: w434 -> [w444 w501]
                          frame True {
                            # "octave: complex"
                            n140 = case shown="Default" w452 {
                              tunnel: w451 -> [w455 w477 w499]
                              tunnel: w450 -> [w454 w476 _]
                              tunnel: [w462 w484 w498] -> w449
                              tunnel: w448 -> [w463 w485 _]
                              tunnel: w447 -> [w460 w482 _]
                              tunnel: w446 -> [w458 w480 _]
                              tunnel: w445 -> [w457 w479 _]
                              tunnel: w444 -> [_ _ w497]
                              frame "single" {
                                # "octave: single real array"
                                n141 = Byte Array To String(unsigned byte array=w454) -> (string=w453:string)
                                n142 = Unflatten From String(type=csg[] [], binary string=w453, data includes array or string size? (T)=FALSE ("prepend array or string size? (T)"), byte order (0:big-endian, network order)=T4."little-endian", error in (no error)=w455) -> (value=w461:csg[], error out=w464:errorcluster)  [unwired: 1 out]
                                n143 = case shown="2" w460 {
                                tunnel: w461 -> [w467 w474]
                                tunnel: [w468 w473] -> w459
                                tunnel: w458 -> [_ w472]
                                tunnel: w457 -> [_ w471]
                                frame Default {
                                # "1D"
                                n144 = To Variant(anything=w467) -> (Variant=w468:variant)
                                }
                                frame 2 {
                                # "2D"
                                n145 = Reshape Array(w474, w472, w471) -> (w470:csg[][])
                                n146 = Transpose 2D Array(2D array=w470) -> (transposed array=w469:csg[][])
                                n147 = To Variant(anything=w469) -> (Variant=w473:variant)
                                }
                                }
                                n148 = property class="Ctl"(reference=w463, error in=w464, "Value"=w459) -> (error out=w462:errorcluster)  [unwired: 1 out]
                              }
                              frame "double" {
                                # "octave: double real array"
                                n149 = Byte Array To String(unsigned byte array=w476) -> (string=w475:string)
                                n150 = Unflatten From String(type=cdb[] [], binary string=w475, data includes array or string size? (T)=FALSE ("prepend array or string size? (T)"), byte order (0:big-endian, network order)=T4."little-endian", error in (no error)=w477) -> (value=w483:cdb[], error out=w486:errorcluster)  [unwired: 1 out]
                                n151 = case shown="2" w482 {
                                tunnel: w483 -> [w489 w496]
                                tunnel: [w490 w495] -> w481
                                tunnel: w480 -> [_ w494]
                                tunnel: w479 -> [_ w493]
                                frame Default {
                                # "1D"
                                n152 = To Variant(anything=w489) -> (Variant=w490:variant)
                                }
                                frame 2 {
                                # "2D"
                                n153 = Reshape Array(w496, w494, w493) -> (w492:cdb[][])
                                n154 = Transpose 2D Array(2D array=w492) -> (transposed array=w491:cdb[][])
                                n155 = To Variant(anything=w491) -> (Variant=w495:variant)
                                }
                                }
                                n156 = property class="Ctl"(reference=w485, error in=w486, "Value"=w481) -> (error out=w484:errorcluster)  [unwired: 1 out]
                              }
                              frame Default {
                                # "error: invalid octave data"
                                n157 = call "Generate Custom Error.vi"("error in"=w499, "PAR1"=w497, "GOLPI error"=Custom_Error_Codes_Enum_Type_Def.vi."98 internal error") -> ("error out"=w498:errorcluster)  [unwired: 8 in]
                              }
                            }
                          }
                          frame False {
                            # "not allowed reals"
                            n158 = call "Generate Custom Error.vi"("error in"=w503, "PAR1"=w501, "GOLPI error"=Custom_Error_Codes_Enum_Type_Def.vi."83 struct: type mismatch of PAR1") -> ("error out"=w502:errorcluster)  [unwired: 8 in]
                          }
                        }
                      }
                      frame 80 {
                        w506 = u32 1 ("Number of Columns")
                        w522 = refnum<vi> refnum  # Array
                        # "restore original visible size"
                        # "set visible array size to [1,1]\n#todo: probably unnecessary\nbut without this indexing never works\nas it shoudl, it sometimes writes to [+1;+1] offset"
                        # "cast ref to general array"
                        # "clear array first\n#todo: this is fucked up way\nbecause it may have some \ndata as default but I found\nno better way"
                        # "lv: cluster"
                        n159 = To More Specific Class(target class=w522, reference=w524, error in=w523) -> (specific class reference=w516:refnum<vi>, error out=w517:errorcluster)
                        n160 = invoke class="Arr" method="Reinit To Default"(reference=w516, error in=w517) -> (reference out=w514:refnum<vi>, error out=w515:errorcluster)  [unwired: 1 in, 1 out]
                        n161 = property class="Arr"(reference=w514, error in=w515, "Number of Columns"=w506, "Number of Rows"=w506) -> (reference out=w507:refnum<vi>, error out=w513:errorcluster, "Number of Columns"=w509:u32, "Number of Rows"=w508:u32)
                        n162 = case shown="Default" w510 {
                          tunnel: [w529 w549 w572] -> w512
                          tunnel: w521 -> [w528 w548 _]
                          tunnel: w520 -> [w525 w547 _]
                          tunnel: w519 -> [_ w546 _]
                          tunnel: w518 -> [_ w545 _]
                          tunnel: w513 -> [w527 w543 w571]
                          tunnel: w507 -> [w526 w542 _]
                          tunnel: w505 -> [_ _ w570]
                          frame 1 {
                            # "1D array"
                            n163 = for {
                              tunnel: w526 -> [w537]
                              shift-right: [w534] -> w529
                              shift-left: w527 -> [w538]
                              tunnel: w528 -> [w532]
                              tunnel: w525 -> [w531] mode=indexing
                              i -> [w530]
                              w540 = refnum<vi> refnum  # Cluster
                              n164 = Build Array(w530) -> (w536:i32[])
                              n165 = property class="Arr"(reference=w537, error in=w538, "Index Values"=w536) -> (error out=w541:errorcluster, "Array Element"=w539:refnum<vi>)  [unwired: 1 out]
                              n166 = To More Specific Class(target class=w540, reference=w539, error in=w541) -> (specific class reference=w533:refnum<vi>, error out=w535:errorcluster)
                              n167 = call "Struct Fill Cluster By Items Record.vi"("error in"=w535, "data start offset (0)"=w531, "data in"=w532, "cluster ref (empty)"=w533) -> ("error out"=w534:errorcluster)  [unwired: 5 in, 2 out]
                            }
                          }
                          frame 2 {
                            # "2D array"
                            n168 = Reshape Array(w547, w545, w546) -> (w544:u32[][])
                            n169 = for {
                              tunnel: w542 -> [w555]
                              shift-right: [w554] -> w549
                              shift-left: w543 -> [w553]
                              tunnel: w548 -> [w551]
                              tunnel: w544 -> [w550] mode=indexing
                              i -> [w552]
                              n170 = for {
                                tunnel: w555 -> [w565]
                                shift-right: [w562] -> w554
                                shift-left: w553 -> [w566]
                                tunnel: w552 -> [w557]
                                tunnel: w551 -> [w560]
                                tunnel: w550 -> [w559] mode=indexing
                                i -> [w558]
                                w568 = refnum<vi> refnum  # Cluster
                                n171 = Build Array(w558, w557) -> (w564:i32[])
                                n172 = property class="Arr"(reference=w565, error in=w566, "Index Values"=w564) -> (error out=w569:errorcluster, "Array Element"=w567:refnum<vi>)  [unwired: 1 out]
                                n173 = To More Specific Class(target class=w568, reference=w567, error in=w569) -> (specific class reference=w561:refnum<vi>, error out=w563:errorcluster)
                                n174 = call "Struct Fill Cluster By Items Record.vi"("reinit cluster to default (false)"=FALSE, "error in"=w563, "data start offset (0)"=w559, "data in"=w560, "cluster ref (empty)"=w561) -> ("error out"=w562:errorcluster)  [unwired: 4 in, 2 out]
                              }
                            }
                          }
                          frame Default {
                            # "fail: invalid dimensions"
                            n175 = call "Generate Custom Error.vi"("error in"=w571, "PAR1"=w570, "GOLPI error"=Custom_Error_Codes_Enum_Type_Def.vi."98 internal error") -> ("error out"=w572:errorcluster)  [unwired: 8 in]
                          }
                        }
                        n176 = property class="Arr"(reference=w507, error in=w512, "Number of Columns"=w509, "Number of Rows"=w508) -> (error out=w511:errorcluster)  [unwired: 1 out]
                      }
                      frame 48, 50 {
                        w584 = refnum<vi> refnum  # Array
                        # "cast ref to general array"
                        # "lv: some kind of string"
                        n177 = To More Specific Class(target class=w584, reference=w586, error in=w585) -> (specific class reference=w579:refnum<vi>, error out=w580:errorcluster)
                        n178 = Multiply(x=w578, y=w577) -> (x*y=w576:i32)
                        n179 = case shown="Default" w581 {
                          selector: w581 -> [w593 _]
                          tunnel: [w591 w665] -> w574
                          tunnel: w583 -> [w601 _]
                          tunnel: w582 -> [w600 _]
                          tunnel: w577 -> [w599 _]
                          tunnel: w578 -> [w598 _]
                          tunnel: w580 -> [w596 w664]
                          tunnel: w579 -> [w590 _]
                          tunnel: w576 -> [w588 _]
                          tunnel: w575 -> [w587 _]
                          frame 1, 2 {
                            # "fail?"
                            # "1D/2D array - extract string array from octave data"
                            n180 = Reshape Array(w600, w598, w599) -> (w597:u32[][])
                            n181 = for {
                              shift-right: [w646] -> w592
                              shift-left: w596 -> [w645]
                              tunnel: w601 -> [w644]
                              tunnel: w597 -> [w643] mode=indexing
                              tunnel: [w642] -> w589 mode=indexing
                              tunnel: [w641] -> w595 mode=indexing
                              n182 = for {
                                shift-right: [w660] -> w646
                                shift-left: w645 -> [w663]
                                tunnel: w644 -> [w662]
                                tunnel: w643 -> [w661] mode=indexing
                                tunnel: [w656] -> w642 mode=indexing if=w647
                                tunnel: [w647] -> w641 mode=indexing
                                # "extract item of array"
                                # "item is part of cell array of strings"
                                n183 = call "Struct Parse Binary.vi"("error in"=w663, "data start offset (0)"=w661, "data in"=w662) -> ("error out"=w660:errorcluster, "struct items"=w659:T1[])  [unwired: 7 in]
                                n184 = Array Size(array=w659) -> (size(s)=w654:i32)
                                n185 = Index Array(array=w659) -> (element=w658:T1)  [unwired: 1 in]
                                n186 = Equal?(x=w654, y=1) -> (x = y?=w650:bool)
                                n187 = Unbundle By Name(w658) -> ("data"=w657:u8[], "name"=w651:string, "type"=w652:T2)
                                n188 = Byte Array To String(unsigned byte array=w657) -> (string=w656:string)
                                n189 = Empty String/Path?(string/path=w651) -> (empty?=w649:bool)
                                n190 = Equal?(x=w652, y=Struct_Item_Types."string") -> (x = y?=w648:bool)
                                n191 = Compound Arithmetic op=AND(w649, w648, w650) -> (w647:bool)
                              }
                            }
                            n192 = And Array Elements(Boolean array=w595) -> (logical AND=w594:bool)
                            n193 = case shown="True" w594 {
                              tunnel: w593 -> [_ w609]
                              tunnel: w592 -> [w602 w608]
                              tunnel: [w602 w607] -> w591
                              tunnel: w590 -> [_ w606]
                              tunnel: w589 -> [_ w605]
                              tunnel: w588 -> [_ w604]
                              tunnel: w587 -> [_ w603]
                              frame False {
                                # "fail - some items are not strings!"
                              }
                              frame True {
                                # "oukej - all items are strings"
                                n194 = case shown="1, Default" w609 {
                                tunnel: w608 -> [w616 w631]
                                tunnel: [w615 w630] -> w607
                                tunnel: w606 -> [w614 w629]
                                tunnel: w605 -> [w613 w627]
                                tunnel: w604 -> [w612 _]
                                tunnel: w603 -> [w610 w628]
                                frame 1, Default {
                                # "1D"
                                n195 = Reshape Array(w613, w612) -> (w611:string[])
                                n196 = case shown="32" w610 {
                                tunnel: w616 -> [w620 w625]
                                tunnel: [w619 w624] -> w615
                                tunnel: w614 -> [w618 w623]
                                tunnel: w611 -> [w617 w622]
                                frame Default {
                                # "string"
                                n197 = property class="Arr"(reference=w618, error in=w620, "Value"=w617) -> (error out=w619:errorcluster)  [unwired: 1 out]
                                }
                                frame 50 {
                                # "path"
                                n198 = String To Path(string=w622) -> (path=w621:path[])
                                n199 = property class="Arr"(reference=w623, error in=w625, "Value"=w621) -> (error out=w624:errorcluster)  [unwired: 1 out]
                                }
                                }
                                }
                                frame 2 {
                                # "2D"
                                n200 = Transpose 2D Array(2D array=w627) -> (transposed array=w626:string[][])
                                n201 = case shown="32" w628 {
                                tunnel: w631 -> [w635 w640]
                                tunnel: [w634 w639] -> w630
                                tunnel: w629 -> [w633 w638]
                                tunnel: w626 -> [w632 w637]
                                frame Default {
                                # "string"
                                n202 = property class="Arr"(reference=w633, error in=w635, "Value"=w632) -> (error out=w634:errorcluster)  [unwired: 1 out]
                                }
                                frame 50 {
                                # "path"
                                n203 = String To Path(string=w637) -> (path=w636:path[][])
                                n204 = property class="Arr"(reference=w638, error in=w640, "Value"=w636) -> (error out=w639:errorcluster)  [unwired: 1 out]
                                }
                                }
                                }
                                }
                              }
                            }
                          }
                          frame Default {
                            # "fail: invalid dimensions"
                            n205 = call "Generate Custom Error.vi"("error in"=w664, "GOLPI error"=Custom_Error_Codes_Enum_Type_Def.vi."98 internal error") -> ("error out"=w665:errorcluster)  [unwired: 9 in]
                          }
                        }
                      }
                      frame Default {
                        # "invalid lv item type"
                        n206 = call "Generate Custom Error.vi"("error in"=w668, "PAR1"=w667, "GOLPI error"=Custom_Error_Codes_Enum_Type_Def.vi."80 struct: cluster elem. PAR1 not implem.") -> ("error out"=w669:errorcluster)  [unwired: 8 in]
                      }
                    }
                  }
                }
              }
              frame "Cluster" {
                # "cluster"
                n207 = Equal?(x=w680, y=1) -> (x = y?=w675:bool)
                n208 = Equal?(x=w678, y=Struct_Item_Types."cell array") -> (x = y?=w676:bool)
                n209 = Compound Arithmetic op=AND(w675, w676) -> (w674:bool)
                n210 = case shown="False" w674 {
                  tunnel: w681 -> [w683 w690]
                  tunnel: w673 -> [_ w685]
                  tunnel: w672 -> [_ w688]
                  tunnel: [w682 w687] -> w671
                  frame False {
                    # "invalid octave data"
                    n211 = call "Generate Custom Error.vi"("error in"=w683, "GOLPI error"=Custom_Error_Codes_Enum_Type_Def.vi."81 struct: structure field PAR1 not implem.") -> ("error out"=w682:errorcluster)  [unwired: 9 in]
                  }
                  frame True {
                    w691 = refnum<vi> refnum  # Cluster
                    # "!!! recursion !!!"
                    # "convert ctrl ref\nto cluster ref"
                    # "octave: struct or cell array with one elemnt which is struct"
                    n212 = To More Specific Class(target class=w691, reference=w685, error in=w690) -> (specific class reference=w686:refnum<vi>, error out=w689:errorcluster)
                    n213 = call "Struct Fill Cluster By Items Record.vi"("error in"=w689, "data in"=w688, "cluster ref (empty)"=w686) -> ("error out"=w687:errorcluster)  [unwired: 6 in, 2 out]
                  }
                }
              }
              frame Default {
                # "unknown class of elemenet of cluster"
                n214 = call "Generate Custom Error.vi"("error in"=w693, "PAR1"=w694, "GOLPI error"=Custom_Error_Codes_Enum_Type_Def.vi."80 struct: cluster elem. PAR1 not implem.") -> ("error out"=w692:errorcluster)  [unwired: 8 in]
              }
            }
          }
          frame -1 {
            # "structure field NOT found in cluster fields, nothing to do here"
          }
        }
      }
    }
  }
  "error out" <- w9
  "cluster ref out (copy)" <- "cluster ref (empty)"
